vi "elevator 全局变量.vi"() -> ()   [LabVIEW 2016, in "elevator.lvlib"]
uses:
  elevator.lvlib
  <vilib>/Plasmionique/MB Master/MB_Master/MB_Master.lvclass
panel:
  in  "编码器工程量转换":cluster{"编码器计数值":dbl, "工程计量值":dbl}={"编码器计数值"=1.0, "工程计量值"=1.0}
  out "编码器工程值":sgl
  in  "编码器计数值":i32
  in  "MB session in":refnum<class "MB_Master.lvclass">
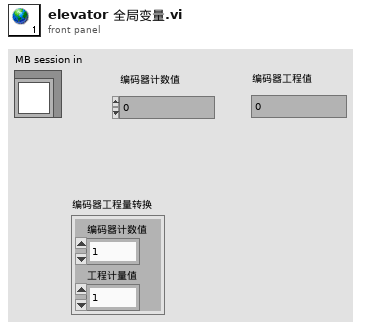
[diagram p1: front panel]
diagram:
